vi "Scope DPO Save Recall.vi"(8 "error in (no error)":errorcluster, 9 "Location":u16(ring)=1 items=["Location 1"=1, "Location 2"=2, "Location 3"=3, "Location 4"=4, "Location 5"=5, "Location 6"=6, "Location 7"=7, "Location 8"=8, "Location 9"=9, "Location 10"=10], 10 "Save/Recal":u16(ring) items=["Save", "Recall"], 11 "VISA In":refnum<visa-resource-name>) -> (0 "error out":errorcluster, 3 "VISA Out":refnum<visa-resource-name>)   [LabVIEW 2012]
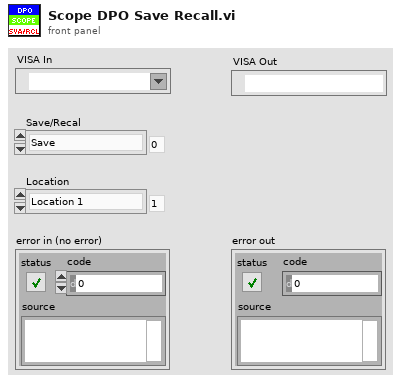
[diagram p1: front panel]
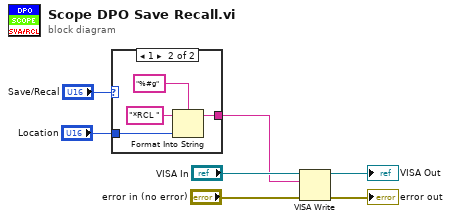
[diagram p0: block diagram]
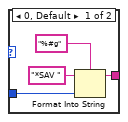
[diagram p2: hidden frame]
diagram:
  n1 = case shown="1" "Save/Recal" {
    tunnel: "Location" -> [w9 w12]
    tunnel: [w8 w13] -> w1
    frame 0, Default {
      n2 = Format Into String(format string="%#g", initial string="*SAV ", w9) -> (resulting string=w8:string)  [unwired: 1 in, 1 out]
    }
    frame 1 {
      n3 = Format Into String(format string="%#g", initial string="*RCL ", w12) -> (resulting string=w13:string)  [unwired: 1 in, 1 out]
    }
  }
  n4 = VISA Write(VISA resource name="VISA In", write buffer=w1, error in (no error)="error in (no error)") -> (VISA resource name out=→"VISA Out":refnum<visa-resource-name>, error out=→"error out":errorcluster)  [unwired: 1 out]
